vi "Prax13y2.vi"() -> ()   [LabVIEW 2020]
panel:
  out "Data 1":u32(graph)
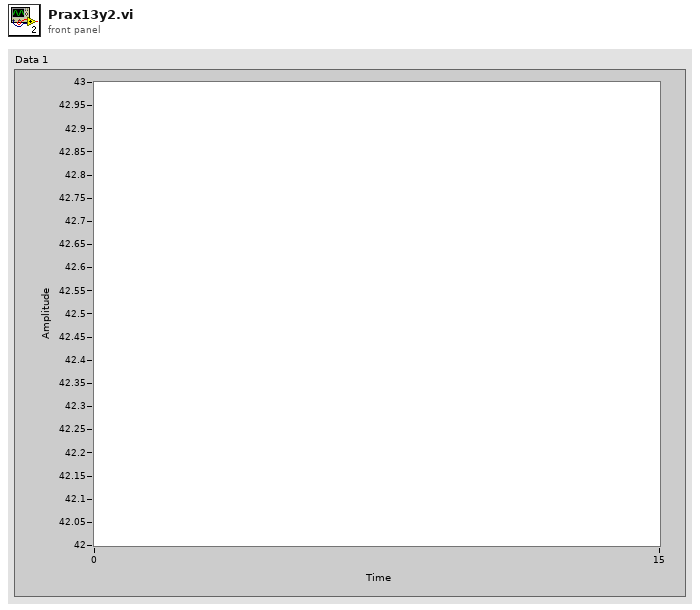
[diagram p1: front panel]
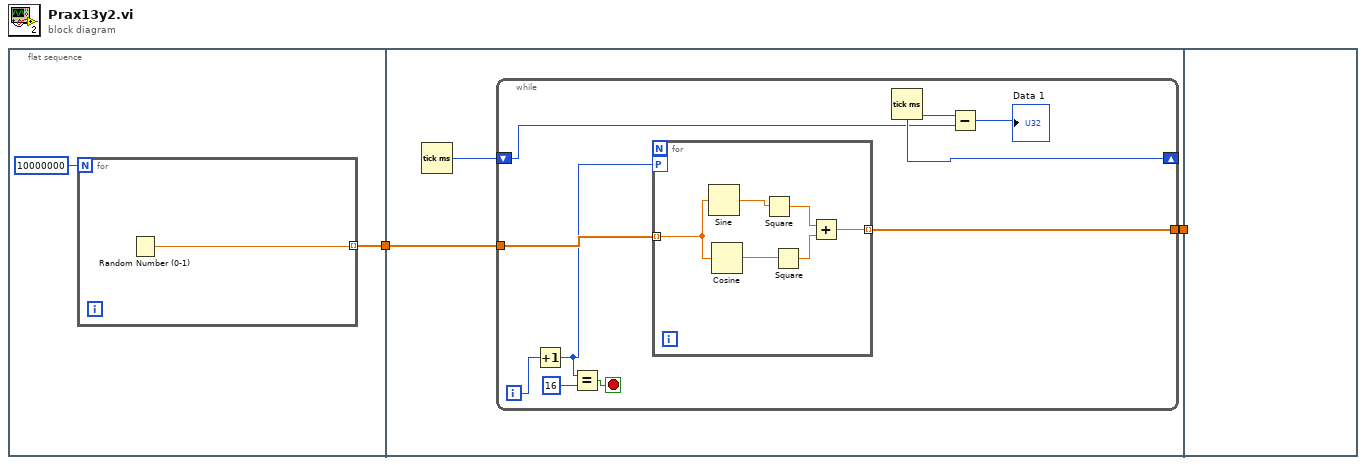
[diagram p0: block diagram]
diagram:
  n1 = flat-sequence {
    tunnel: [w3] -> w2
    tunnel: w2 -> [w8]
    tunnel: [w6] -> w1
    tunnel: w1 -> [_]
    frame #0 {
      n2 = for {
        N: 10000000 -> [_]
        tunnel: [w5] -> w3 mode=indexing
        n3 = Random Number (0-1)() -> (number: 0 to 1=w5:dbl)
      }
    }
    frame #1 {
      n4 = Tick Count (ms)() -> (millisecond timer value=w7:u32)
      n5 = while {
        tunnel: w8 -> [w17]
        shift-right: [w13] -> _
        shift-left: w7 -> [w12]
        tunnel: [w11] -> w6
        i -> [w16]
        stop <- w14 stop-if-true
        n6 = Increment(x=w16) -> (x+1=w10:i32)
        n7 = Equal?(x=w10, y=16) -> (x = y?=w14:bool)
        n8 = for {
          workers-P: w10 -> [_]
          tunnel: [w19] -> w11 mode=indexing
          tunnel: w17 -> [w18] mode=indexing
          n9 = Sine(x=w18) -> (sin(x)=w22:dbl)
          n10 = Cosine(x=w18) -> (cos(x)=w23:dbl)
          n11 = Square(x=w22) -> (x^2=w21:dbl)
          n12 = Square(x=w23) -> (x^2=w20:dbl)
          n13 = Add(x=w21, y=w20) -> (x+y=w19:dbl)
        }
        n14 = Tick Count (ms)() -> (millisecond timer value=w13:u32)
        n15 = Subtract(x=w13, y=w12) -> (x-y=→"Data 1":u32)
      }
    }
    frame #2 {
    }
  }
